vi "Tell Parent.vi"(4 "Priority":bool, 7 "Actor in":refnum<class "Actor.lvclass">, 9 "Error":errorcluster, 10 "Actor":refnum<class "Actor.lvclass">) -> (0 "Error out":errorcluster)   [LabVIEW 2025, in "jettl.lvlib" / "Stopped Msg.lvlib"]
uses:
  Stopped Msg.lvlib
  Actor/Actor.lvclass
  Stopped Msg/Stopped Msg.lvclass
  C:/git/jettl/src/jettl/jettl/Msg/Msg.lvclass
  jettl.lvlib
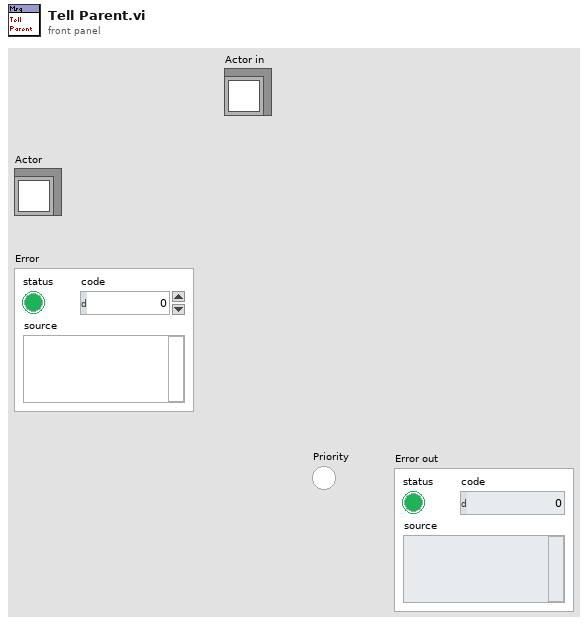
[diagram p1: front panel]
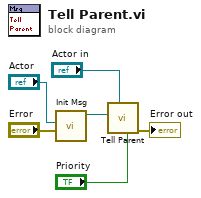
[diagram p0: block diagram]
diagram:
  n1 = call "Init Msg.vi"("Error"="Error", "Actor"="Actor") -> ("Stopped Msg out"=w4:refnum<class "Stopped Msg.lvclass">)  [unwired: 9 in]
  n2 = call "Tell Parent.vi"("Priority"="Priority", "Actor in"="Actor in", "Msg"=w4) -> ("Error out"=→"Error out":errorcluster)  [unwired: 8 in]
